vi "PS90_SimpleConnect.vi"(8 "error in (no error)":errorcluster, 9 "Serial number":string, 10 "Control unit ID":i32=1 min=1 max=20, 11 "DLOwis.lvclass":refnum<class "DLOwis.lvclass">) -> (0 "error out":errorcluster, 3 "DLOwis.lvclass":refnum<class "DLOwis.lvclass">)   [LabVIEW 2018]
doc: "PS90_SimpleConnect.vi, created: 06.10.2006 alex; last change: 18.07.2016 alex;\n\n<B>FUNCTION:</B> \n\nFind control unit with the specified serial number and connect to it.\n*Serial interface (communication via USB or serial port)*\nThe application software can access this interface in the same way as \nit would access a standard serial port (COM). The parameters for Baudrate, \nParity, Databits and Stopbits are predefined (9600, no parity, 8 databits, 1 stopbit).\nThe software handshake character is CR.\n*Ethernet interface (communication via Com-Server)*\nAs Com-Server the OWIS software tool \"OWISerialServer.exe\" may be used\n(..\\OWISoft\\Application\\system). The application software can access \nthis interface via Windows TCP socket: special communication for OWIS software\n(command + delay). The software handshake character is CR.\n----------------------------------------------------------------------------------------\n<B>INPUT:</B>\n[I32] <B>Control unit ID:</B> control unit index 1-10. (Default=1, Range=1...20) \n11...20 - debug mode\n1...10 - standard mode\n[CStr] <B>Serial number:</B> control unit serial number. (Default=empty string)\nUSB or serial port\nempty string - the first found control unit is connected;\n\"12345678\" - control unit with the specified serial number is connected;\nEthernet interface\n\"net\" - control unit is connected to the Com-Server (local application) \nby the first found local IP address and port number 1200.\n[CLU] <B>error in</B>\n----------------------------------------------------------------------------------------\n<B>OUTPUT:</B>\n[CLU] <B>error out</B>\n0 - no error,\n1 - function error (invalid parameters),\n5 - no response from control unit (check cable, connection or reset control unit),\n7 - control unit with the specified serial number is not found,\n9 - no connection to tcp/ip socket.\n----------------------------------------------------------------------------------------\n<B>SUB-VIs:</B>\n----------------------------------------------------------------------------------------\n<B>EXT-Calls:</B>\nps90.dll (V2.00)\n----------------------------------------------------------------------------------------"
uses:
  DLOwis.lvclass
  C:/Users/Sergey Denisov/Documents/REPS/TRANCON/Classes/Delay Line/DelayLine.lvclass
  DelayLine.lvclass/DelayLine.ctl
  DelayLine.lvclass
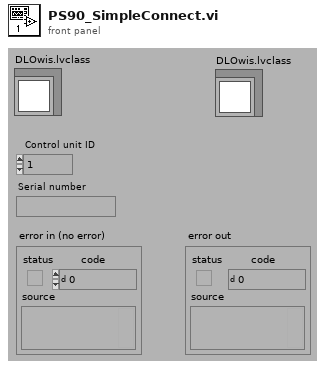
[diagram p1: front panel]
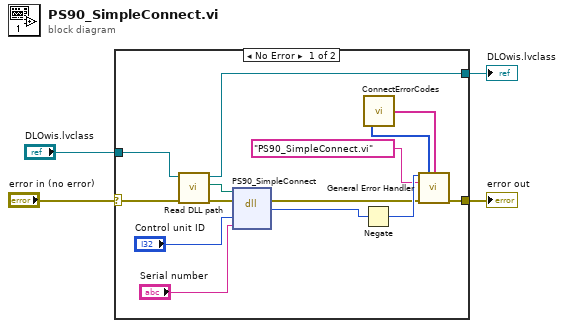
[diagram p0: block diagram]
diagram:
  n1 = case shown="No Error" "error in (no error)" {
    selector: "error in (no error)" -> [w7 w20]
    tunnel: [w17 w20] -> w4
    tunnel: [w5 w19] -> w2
    tunnel: "DLOwis.lvclass" -> [w10 w19]
    frame No Error {
      n2 = call "Read DLL path.vi"("error in (no error)"=w7, "DelayLine in"=w10) -> ("error out"=w9:errorcluster, "DLL path"=w6:path, "DelayLine out"=w5:refnum<class "DLOwis.lvclass">)  [unwired: 7 in]
      n3 = dll-call lib="C:/Users/Sergey Denisov/Documents/REPS/TRANCON/DLL/ps90.dll" fn="PS90_SimpleConnect"(path in=w6, error in=w9, "Index"="Control unit ID", "szSerNum"="Serial number") -> (error out=w8:errorcluster, "Rückgabetyp"=w16:i32)  [unwired: 3 in, 1 out]
      n4 = Negate(x=w16) -> (-x=w14:i32)
      n5 = call "ConnectErrorCodes.vi"() -> ("[user-defined descriptions]"=w11:string[], "[user-defined codes]"=w12:i32[])
      n6 = call <vilib>:"General Error Handler.vi"("[error code] (0)"=w14, "[user-defined codes]"=w12, "[user-defined descriptions]"=w11, "[error source] (\" \")"="PS90_SimpleConnect.vi", "error in (no error)"=w8) -> ("error out"=w17:errorcluster)  [unwired: 6 in, 4 out]
    }
    frame Error {
    }
  }
  "error out" <- w4
  "DLOwis.lvclass" <- w2
